vi "resCalc.vi"(10 "Frequency Sweep":dbl[](array[numeric]), 11 "Start F, Hz (1355)":i32=1355) -> (2 "F-res, Hz":dbl, 3 "Frequency Scan":cluster{i32[], "Best Gaussian Fit":dbl[]}[](graph))   [LabVIEW 2011]
uses:
  <vilib>/Analysis/6fits.llb/Curve Fitting Criteria.ctl
  <vilib>/Analysis/3filter.llb/Savitzky-Golay Filter (DBL).vi
  <vilib>/Analysis/NI_AALPro.lvlib
  <vilib>/Analysis/NI_AALBase.lvlib
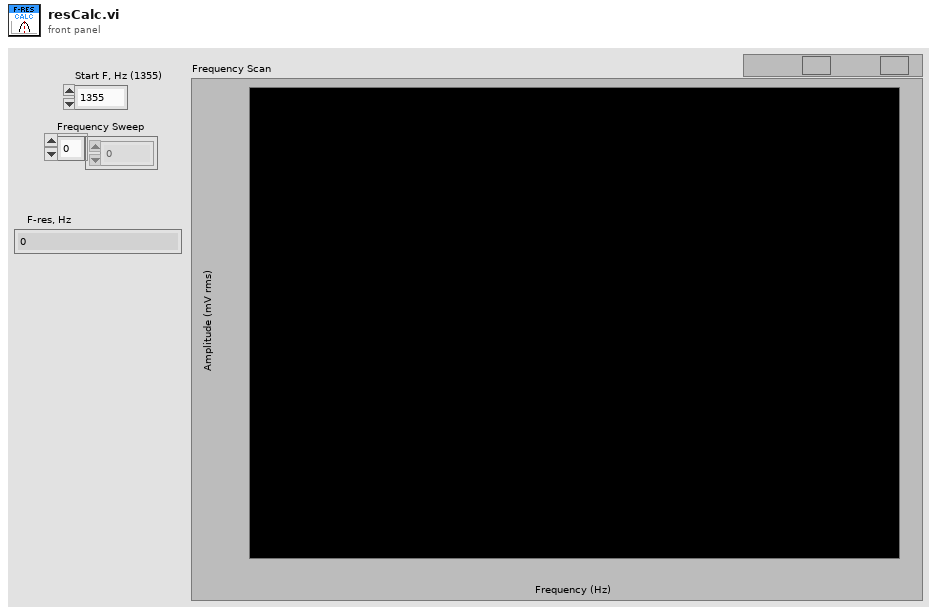
[diagram p1: front panel]
types:
  T1 = typedef "NI_AALPro.lvlib/Curve Fitting Criteria.ctl" = u16
  T2 = cluster{"Array":i32[], "Best Gaussian Fit":dbl[]}
  T3 = cluster{"Array":i32[], "Best Gaussian Fit":dbl[]}[]
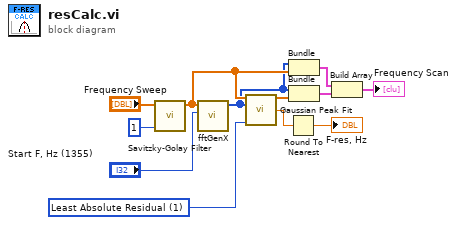
[diagram p0: block diagram]
diagram:
  w10 = T1 1 items=["Least Square", "Least Absolute Residual", "Bisquare"] ("method")
  n1 = call-poly <vilib>:"Savitzky-Golay Filter.vi"("polynomial order"=1, "X"="Frequency Sweep") -> ("Filtered X"=w9:dbl[])  [unwired: 8 in, 1 out]
  n2 = call "fftGenX.vi"("start"="Start F, Hz (1355)", "Output Array"=w9) -> ("Array"=w6:i32[])  [unwired: 9 in]
  n3 = call <vilib>:"Gaussian Peak Fit.vi"("Y"=w9, "X"=w6, "method"=w10) -> ("Best Gaussian Fit"=w4:dbl[], "center"=w5:dbl)  [unwired: 6 in, 5 out]
  n4 = Round To Nearest(number=w5) -> (nearest integer value=→"F-res, Hz":dbl)
  n5 = Bundle("Array"=w6, "Filtered X"=w9) -> (w2:cluster{"Array":i32[], "Filtered X":dbl[]})  [unwired: 1 in]
  n6 = Bundle("Array"=w6, "Best Gaussian Fit"=w4) -> (w7:T2)  [unwired: 1 in]
  n7 = Build Array(w2, w7) -> (→"Frequency Scan":T3)
